vi "Receive Message.vi"(6 "priority":i32, 10 "LoggedActor in":refnum<class "LoggedActor.lvclass">, 11 "Message in":refnum<class "Message.lvclass">) -> (0 "error out":errorcluster, 2 "Actor out":refnum<class "Actor.lvclass">)   [LabVIEW 2020, in "LoggedActor.lvclass"]
doc: "This VI should be overriden ONLY if you are creating a proxy actor for remote transmission. If you are, override this VI to transmit the received message to a new destination, maintaining the given priority."
uses:
  <vilib>/gpm_packages/@cs/Network-interface/Source/Logged Actor/LoggedActor.lvclass
  <vilib>/ActorFramework/Message/Message.lvclass
  <vilib>/ActorFramework/Actor/Actor.lvclass
  <vilib>/gpm_packages/@cs/event-logger/Source/Composed Log/Types/Log Level.ctl
  <vilib>/gpm_packages/@cs/event-logger/Source/Composed Log/Composed Log.lvlib
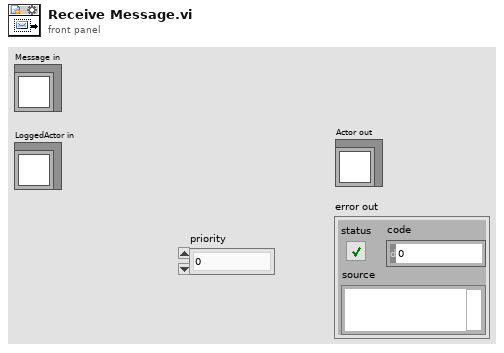
[diagram p1: front panel]
types:
  T1 = typedef "Composed Log.lvlib/Log Level.ctl" = enum16{"Debug", "Info", "Warning", "Error", "Critical"}
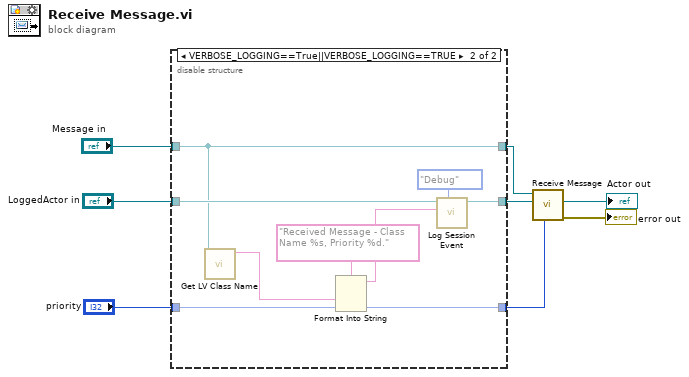
[diagram p0: block diagram]
diagram:
  n1 = disable-structure shown="VERBOSE_LOGGING==True||VERBOSE_LOGGING==TRUE" {
    disable-tunnel: "Message in" -> [w9 w15]
    disable-tunnel: "LoggedActor in" -> [w10 w19]
    disable-tunnel: "priority" -> [w11 w16]
    disable-tunnel: [w11 w16] -> w3
    disable-tunnel: [w10 w18] -> w2
    disable-tunnel: [w9 w15] -> w1
    frame condition #0 (active) {
    }
    frame condition #1 {
      n2 = call <vilib>:"Get LV Class Name.vi"("object"=w15) -> ("class name"=w12:string)  [unwired: 9 in, 1 out]
      n3 = Format Into String(format string="Received Message - Class Name %s, Priority %d.", w12, w16) -> (resulting string=w14:string)  [unwired: 2 in, 1 out]
      n4 = call <vilib>:"Log Session Event.vi"("Event Level"=Log_Level."Debug", "Event Data"=w14, "SessionActor in"=w19) -> ("SessionActor out"=w18:refnum<class "LoggedActor.lvclass">)  [unwired: 7 in, 1 out]
    }
  }
  n5 = call-parent "Receive Message.vi"("priority"=w3, "Actor in"=w2, "Message in"=w1) -> ("error out"=→"error out":errorcluster, "Actor out"=→"Actor out":refnum<class "Actor.lvclass">)  [unwired: 7 in]
